vi "Fetch Single Record Multiple Channel(Wfm).vi"(5 "FIFO Type":T1=enum."Fast FIFO", 7 "Timeout (s)":i32=5, 8 "error in":errorcluster, 11 "FPGA VI Reference In":refnum<k20>) -> (0 "error out":errorcluster, 2 "Acquired Data":waveform(dbl)[](array[waveform]), 3 "FPGA VI Reference Out":refnum<k20>)   [LabVIEW 2012]
uses:
  <userlib>/FlexRIO Host Library/FlexRIO Host API/Acquire/FIFO Type.ctl
  <userlib>/FlexRIO Host Library/FlexRIO Host API/Acquire/Fetch/Fetch Acquired Data (U64).vi
  <vilib>/Utility/error.llb/Error Cluster From Error Code.vi
  <vilib>/rvi/errors/niLvFpgaAdjustHostInterfaceError.vi
  <vilib>/rvi/interface/nirviReadWriteControl/nirviReadWriteControl.xnode
  <userlib>/FlexRIO Host Library/FlexRIO Host Library (User).lvlib
  NiFpgaLv.dll
  <vilib>/rvi/interface/Simulation/niFpgaSimulationCallBeginRW.vi
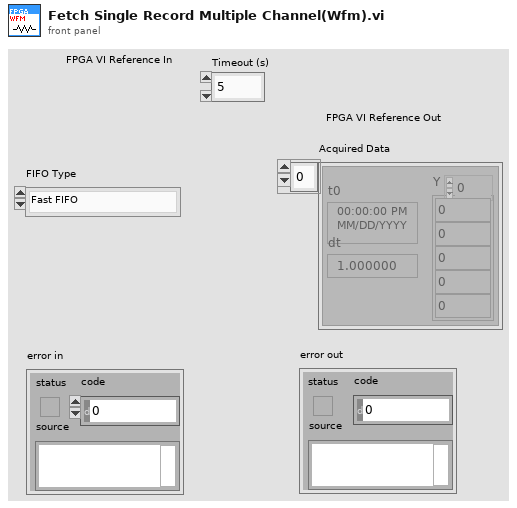
[diagram p1: front panel]
types:
  T1 = typedef "FIFO Type.ctl" = enum16{"FPGA to Host FIFO (U64)", "Generic", "FPGA to Host FIFO (U32)", "Fast FIFO"}
  T2 = cluster{"Load Record Parameters?":bool, "Pre Trigger Samples":u16, "Samples per Record":u16, "Trigger Hold Off":u16, "Record Count":u16}
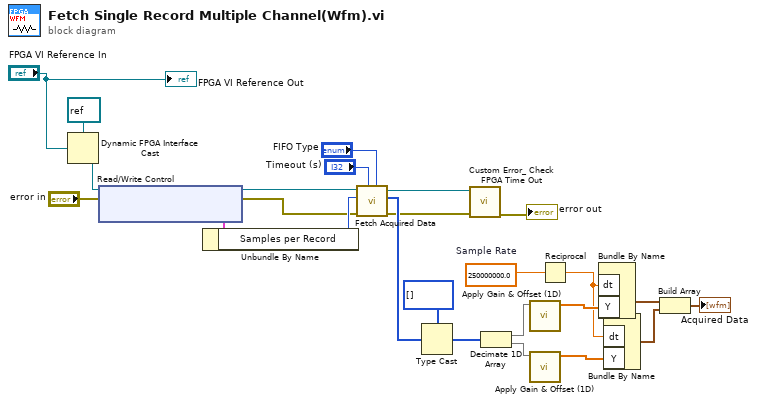
[diagram p0: block diagram]
diagram:
  w3 = 250000000.0  # Sample Rate
  n1 = Dynamic FPGA Interface Cast(Session In=refnum<k20> refnum ("Type"), Type="FPGA VI Reference In") -> (Session Out=w22:refnum<k20>)
  n2 = xnode "Read/Write Control"("FPGA VI Reference In"=w22, "error in"="error in") -> ("FPGA VI Reference Out"=w19:refnum<k20>, "error out"=w18:errorcluster, "Record Parameters"=w21:T2)
  n3 = Unbundle By Name(w21) -> ("Samples per Record"=w20:u16)
  n4 = call-poly <userlib>:"Fetch Acquired Data.vi"("FIFO Type"="FIFO Type", "Timeout (s)"="Timeout (s)", "error out"=w18, "Samples"=w20, "FPGA Reference In"=w19) -> ("error out"=w12:errorcluster, "Data"=w15:u64[], "FPGA Reference Out"=w13:refnum<k20>)  [unwired: 3 in, 1 out]
  n5 = Type Cast(type=i16[] [], x=w15) -> (*(type *) &x=w16:i16[])
  n6 = call <userlib>:"Custom Error_ Check FPGA Time Out.vi"("error in"=w12, "FPGA VI Reference In"=w13) -> ("error out"=→"error out":errorcluster)  [unwired: 8 in, 1 out]
  n7 = Decimate 1D Array(w16) -> (w10:i16[], w9:i16[])
  n8 = call <userlib>:"Apply Gain & Offset (1D).vi"("Raw Data"=w10) -> ("Scaled Data"=w8:dbl[])  [unwired: 10 in]
  n9 = call <userlib>:"Apply Gain & Offset (1D).vi"("Raw Data"=w9) -> ("Scaled Data"=w7:dbl[])  [unwired: 10 in]
  n10 = Reciprocal(x=w3) -> (1/x=w2:dbl)
  n11 = Bundle By Name("dt"=w2, "Y"=w8) -> (w6:waveform(dbl))  [unwired: 1 in]
  n12 = Bundle By Name("dt"=w2, "Y"=w7) -> (w5:waveform(dbl))  [unwired: 1 in]
  n13 = Build Array(w6, w5) -> (→"Acquired Data":waveform(dbl)[])
  "FPGA VI Reference Out" <- "FPGA VI Reference In"
